vi "test-Encrypt (none).vi"(8 "error in (no error)":errorcluster, 11 "TestCase in":refnum<class "Test Argument Encryption.lvclass">) -> (0 "error out":errorcluster, 3 "TestCase out":refnum<class "Test Argument Encryption.lvclass">)   [LabVIEW 2019, in "Test Argument Encryption.lvclass"]
uses:
  Test Argument Encryption.lvclass
  C:/Program Files/National Instruments/LabVIEW 2024/vi.lib/Astemes/LUnit/Test Case.lvclass
  Encryption/Encryption.lvclass
  <vilib>/Astemes/LUnit/Test Case.lvclass/Test Case.ctl
  337534ae-7745-4f7b-a2ba-0ab9d21856e9.vi
  <vilib>/Astemes/LUnit/Core/LUnit Test Case/Private/Append Pass Result.vi
  <vilib>/Astemes/LUnit/Core/LUnit Test Case/Private/Append Fail Result.vi
  337534ae-7745-4f7b-a2ba-0ab9d21856e9.vi/9c5d11cd-9439-4240-a1ee-d9baace9c924.vi
  <vilib>/Astemes/LUnit/Core/LUnit Test Case/Private/Run In UI.vi
  <vilib>/Utility/error.llb/Clear Errors.vi
  Layouts/Layout.lvclass
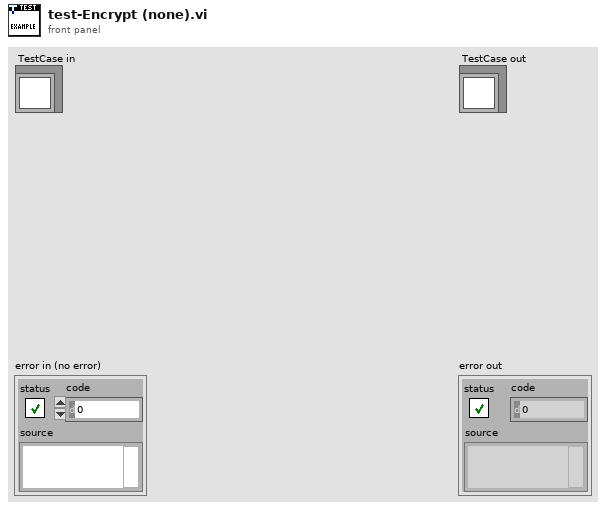
[diagram p1: front panel]
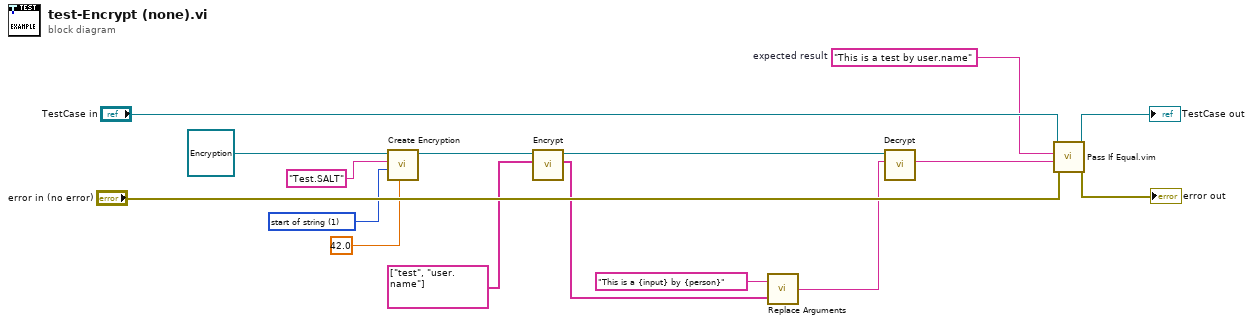
[diagram p0: block diagram]
diagram:
  w9 = u16 1 items=["both", "start of string", "end of string"] ("SALT location (start of string)")
  w12 = "This is a test by user.name"  # expected result
  n1 = call "Create Encryption.vi"("Multiplier"=42.0, "SALT location (start of string)"=w9, "SALT"="Test.SALT", "Encryption Method"=refnum<class "Encryption.lvclass"> refnum ("TSC Event Logger.lvlib:Encryption.lvclass")) -> ("Encryption output"=w7:refnum<class "Encryption.lvclass">)  [unwired: 6 in, 1 out]
  n2 = call-dynamic "Encrypt.vi"("Arguments"=string[] ["test", "user.name"], "Encryption in"=w7) -> ("Encrypted Arguments"=w3:string[], "Encryption out"=w4:refnum<class "Encryption.lvclass">)  [unwired: 7 in, 1 out]
  n3 = call "Replace Arguments.vi"("Arguments"=w3, "Message"="This is a {input} by {person}") -> ("Output Message"=w2:string)
  n4 = call-dynamic "Decrypt.vi"("Message"=w2, "Encryption in"=w4) -> ("Decrypted Message"=w1:string)  [unwired: 7 in, 2 out]
  n5 = call "Pass If Equal.vim"("error in (no error)"="error in (no error)", "Actual"=w1, "Expected"=w12, "LUnit Test Case In"="TestCase in") -> ("error out"=→"error out":errorcluster, "LUnit Test Case Out"=→"TestCase out":refnum<class "Test Argument Encryption.lvclass">)  [unwired: 6 in]
